vi "시리얼_FGV.vi"(8 "Error In":errorcluster caption="에러 입력") -> (0 "Error Out":errorcluster caption="에러 출력")   [LabVIEW 2018]
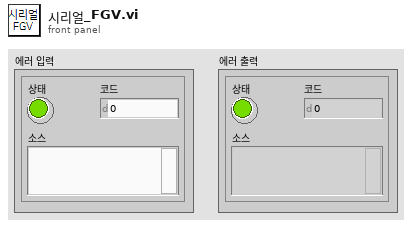
[diagram p1: front panel]
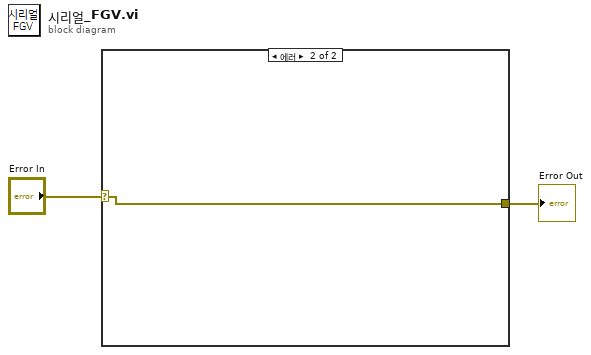
[diagram p0: block diagram]
diagram:
  n1 = case shown="에러" "Error In" {
    selector: "Error In" -> [w3 w4]
    tunnel: [w3 w4] -> w1
    frame No Error {
    }
    frame Error {
    }
  }
  "Error Out" <- w1
